vi "Laurel Serial Item 1 and Item 2.vi"(8 "error in (no error)":errorcluster, 11 "VISA Refnum in":refnum<visa-resource-name>) -> (0 "error out":errorcluster, 1 "Cold Water Rate":dbl, 2 "Cold Water Total":dbl, 3 "VISA Refnum out":refnum<visa-resource-name>)   [LabVIEW 2016]
uses:
  Type Definitions/Laurel Serial Commands.ctl
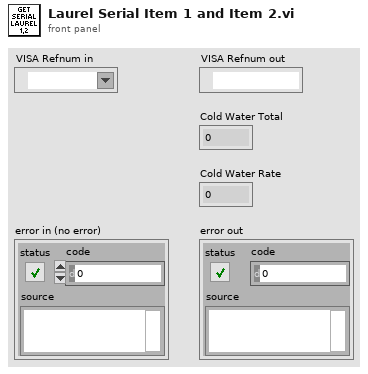
[diagram p1: front panel]
types:
  T1 = typedef "Laurel Serial Commands.ctl" = string
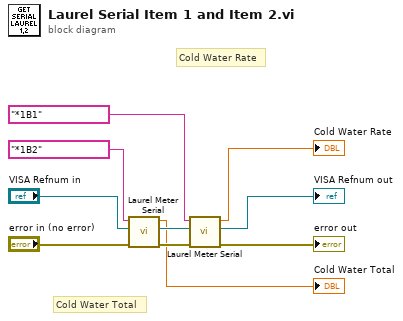
[diagram p0: block diagram]
diagram:
  # "Cold Water Rate"
  # "Cold Water Total"
  n1 = call "Laurel Meter Serial.vi"("error in (no error)"="error in (no error)", "VISA Input"="VISA Refnum in", "Laurel Serial Commands"=T1 "*1B2") -> ("error out"=w6:errorcluster, "VISA Output"=w7:refnum<visa-resource-name>, "Output"=→"Cold Water Total":dbl)  [unwired: 6 in]
  n2 = call "Laurel Meter Serial.vi"("error in (no error)"=w6, "VISA Input"=w7, "Laurel Serial Commands"=T1 "*1B1") -> ("error out"=→"error out":errorcluster, "VISA Output"=→"VISA Refnum out":refnum<visa-resource-name>, "Output"=→"Cold Water Rate":dbl)  [unwired: 6 in]
